vi "ZeroMQ_ReqRep_TCS.vi"() -> ()   [LabVIEW 2018]
uses:
  <vilib>/addons/zeromq/socket_type.ctl
  <vilib>/addons/zeromq/zeromq.lvlib
  <vilib>/addons/zeromq/zmq_socket.lvclass
  <vilib>/addons/zeromq/socket_options.ctl
  <vilib>/addons/zeromq/zmq_context.lvclass
panel:
  out "command":string
  in  "stop 3":bool
  out "error out 3":errorcluster
  out "reply":string
  out "error out 2":errorcluster
  out "message":string
  out "read buffer":string
  in  "stop 2":bool
  out "error out":errorcluster
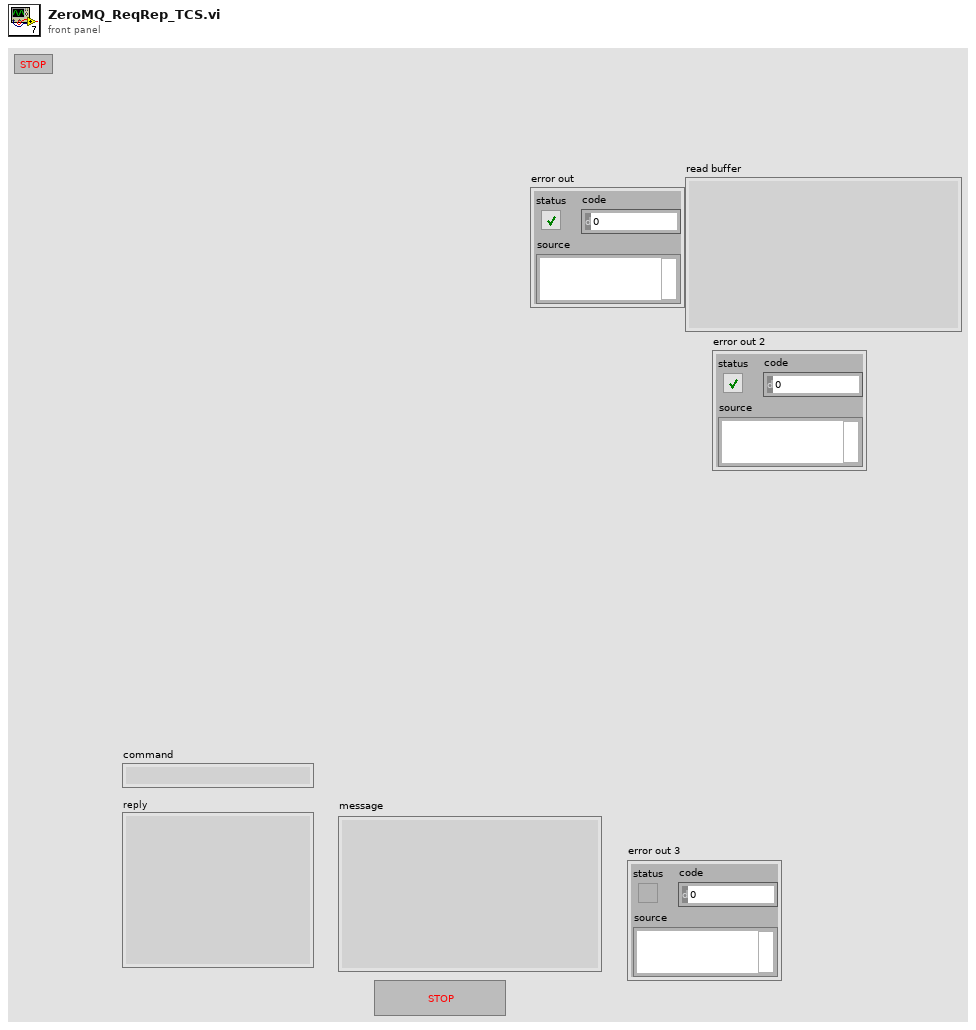
[diagram p1: front panel]
types:
  T1 = typedef "zeromq.lvlib/socket_type.ctl" = enum8{"ZMQ_PAIR", "ZMQ_PUB", "ZMQ_SUB", "ZMQ_REQ", "ZMQ_REP", "ZMQ_DEALER", "ZMQ_ROUTER", "ZMQ_PULL", "ZMQ_PUSH", "ZMQ_XPUB", "ZMQ_XSUB", "ZMQ_STREAM", "ZMQ_SERVER", "ZMQ_CLIENT", "ZMQ_RADIO", "ZMQ_DISH", "ZMQ_GATHER", "ZMQ_SCATTER", "ZMQ_DGRAM"}
  T2 = typedef "zeromq.lvlib/socket_options.ctl" = enum8{"NONE", "ZMQ_HWM", "<2>", "ZMQ_SWAP", "ZMQ_AFFINITY", "ZMQ_ROUTING_ID", "ZMQ_SUBSCRIBE", "ZMQ_UNSUBSCRIBE", "ZMQ_RATE", "ZMQ_RECOVERY_IVL", "ZMQ_MCAST_LOOP", "ZMQ_SNDBUF", "ZMQ_RCVBUF", "ZMQ_RCVMORE", "ZMQ_FD", "ZMQ_EVENTS", "ZMQ_TYPE", "ZMQ_LINGER", "ZMQ_RECONNECT_IVL", "ZMQ_BACKLOG", "ZMQ_RECOVERY_IVL_MSEC", "ZMQ_RECONNECT_IVL_MAX", "ZMQ_MAXMSGSIZE", "ZMQ_SNDHWM", "ZMQ_RCVHWM", "ZMQ_MULTICAST_HOPS", "<26>", "ZMQ_RCVTIMEO", "ZMQ_SNDTIMEO", "<29>", "<30>", "ZMQ_IPV4ONLY", "ZMQ_LAST_ENDPOINT", "ZMQ_ROUTER_MANDATORY", "ZMQ_TCP_KEEPALIVE", "ZMQ_TCP_KEEPALIVE_CNT", "ZMQ_TCP_KEEPALIVE_IDLE", "ZMQ_TCP_KEEPALIVE_INTVL", "ZMQ_TCP_ACCEPT_FILTER", "ZMQ_IMMEDIATE", "ZMQ_XPUB_VERBOSE", "ZMQ_ROUTER_RAW", "ZMQ_IPV6", "ZMQ_MECHANISM", "ZMQ_PLAIN_SERVER", "ZMQ_PLAIN_USERNAME", "ZMQ_PLAIN_PASSWORD", "ZMQ_CURVE_SERVER", "ZMQ_CURVE_PUBLICKEY", "ZMQ_CURVE_SECRETKEY", "ZMQ_CURVE_SERVERKEY", "ZMQ_PROBE_ROUTER", "ZMQ_REQ_CORRELATE", "ZMQ_REQ_RELAXED", "ZMQ_CONFLATE", "ZMQ_ZAP_DOMAIN", "ZMQ_ROUTER_HANDOVER", "ZMQ_TOS", "ZMQ_IPC_FILTER_PID", "ZMQ_IPC_FILTER_UID", "ZMQ_IPC_FILTER_GID", "ZMQ_CONNECT_ROUTING_ID", "ZMQ_GSSAPI_SERVER", "ZMQ_GSSAPI_PRINCIPAL", "ZMQ_GSSAPI_SERVICE_PRINCIPAL", "ZMQ_GSSAPI_PLAINTEXT", "ZMQ_HANDSHAKE_IVL", "<67>", "ZMQ_SOCKS_PROXY", "ZMQ_XPUB_NODROP", "ZMQ_BLOCKY", "ZMQ_XPUB_MANUAL", "ZMQ_XPUB_WELCOME_MSG", "ZMQ_STREAM_NOTIFY", "ZMQ_INVERT_MATCHING", "ZMQ_HEARTBEAT_IVL", "ZMQ_HEARTBEAT_TTL", "ZMQ_HEARTBEAT_TIMEOUT", "ZMQ_XPUB_VERBOSER", "ZMQ_CONNECT_TIMEOUT", "ZMQ_TCP_MAXRT", "ZMQ_THREAD_SAFE", "<82>", "<83>", "ZMQ_MULTICAST_MAXTPDU", "ZMQ_VMCI_BUFFER_SIZE", "ZMQ_VMCI_BUFFER_MIN_SIZE", "ZMQ_VMCI_BUFFER_MAX_SIZE", "ZMQ_VMCI_CONNECT_TIMEOUT", "ZMQ_USE_FD", "ZMQ_GSSAPI_PRINCIPAL_NAMETYPE", "ZMQ_GSSAPI_SERVICE_PRINCIPAL_NAMETYPE", "ZMQ_BINDTODEVICE", "ZMQ_ZAP_ENFORCE_DOMAIN", "ZMQ_LOOPBACK_FASTPATH", "ZMQ_METADATA", "ZMQ_MULTICAST_LOOP", "ZMQ_ROUTER_NOTIFY"}
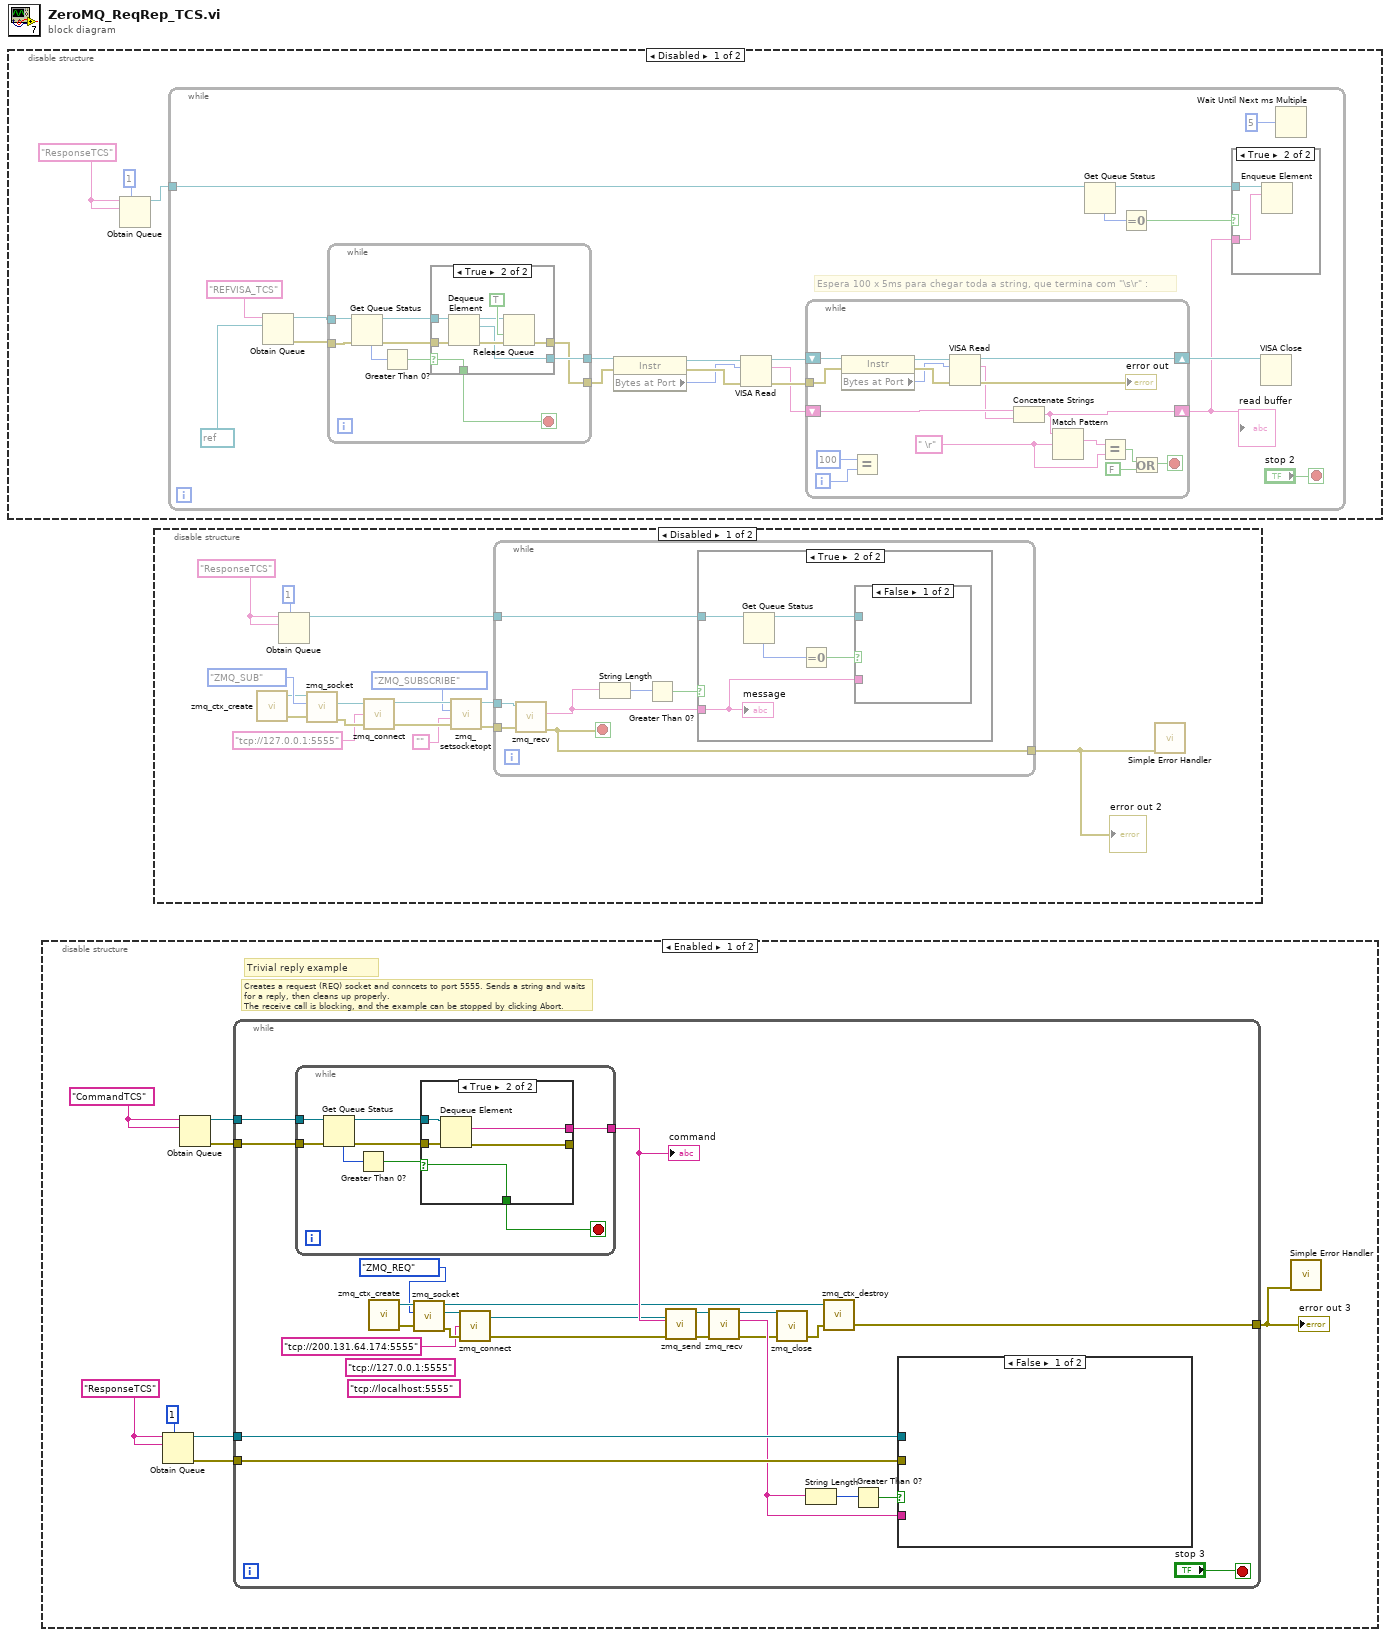
[diagram p0: block diagram]
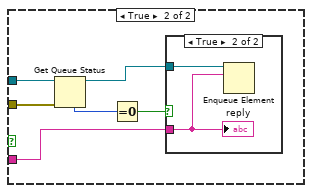
[diagram p2: hidden frame]
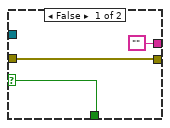
[diagram p4: hidden frame]
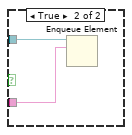
[diagram p7: hidden frame]
diagram:
  n1 = disable-structure shown="Disabled" {
    frame Disabled {
      w3 = "ResponseTCS"
      n2 = Obtain Queue(max queue size (-1, unlimited)=1, name (unnamed)=w3, element data type=w3) -> (queue out=w2:refnum<queue>)  [unwired: 2 in, 2 out]
      n3 = while {
        tunnel: w2 -> [w22]
        stop <- "stop 2" stop-if-true
        # "Espera 100 x 5ms para chegar toda a string, que termina com \"\\s\\r\" :"
        n4 = Obtain Queue(name (unnamed)="REFVISA_TCS", element data type=refnum<visa-resource-name> refnum ("VISA resource name out")) -> (queue out=w18:refnum<queue>, error out=w19:errorcluster)  [unwired: 3 in, 1 out]
        n5 = while {
          tunnel: [w46] -> w8
          tunnel: w18 -> [w45]
          tunnel: w19 -> [w44]
          tunnel: [w43] -> w7
          stop <- w47 stop-if-true
          n6 = Get Queue Status(queue=w45, error in (no error)=w44) -> (queue out=w51:refnum<queue>, error out=w50:errorcluster, # elements in queue=w48:i32)  [unwired: 1 in, 5 out]
          n7 = Greater Than 0?(x=w48) -> (x > 0?=w49:bool)
          n8 = case shown="True" w49 {
            selector: w49 -> [w53 w59]
            tunnel: w51 -> [_ w61]
            tunnel: w50 -> [w52 w60]
            tunnel: [w53 w59] -> w47
            tunnel: [_ w54] -> w46
            tunnel: [w52 w55] -> w43
            frame False {
            }
            frame True {
              n9 = Dequeue Element(queue=w61, error in (no error)=w60) -> (queue out=w57:refnum<queue>, element=w54:refnum<visa-resource-name>, error out=w56:errorcluster)  [unwired: 1 in, 1 out]
              n10 = Release Queue(queue=w57, force destroy? (F)=TRUE, error in (no error)=w56) -> (error out=w55:errorcluster)  [unwired: 2 out]
            }
          }
        }
        n11 = property class="Instr"(reference=w8, error in=w7) -> (reference out=w11:refnum<visa-resource-name>, error out=w10:errorcluster, "Bytes at Port"=w9:u32)
        n12 = VISA Read(VISA resource name=w11, byte count=w9, error in (no error)=w10) -> (VISA resource name out=w5:refnum<visa-resource-name>, read buffer=w4:string, error out=w6:errorcluster)  [unwired: 1 out]
        n13 = while {
          tunnel: w6 -> [w38]
          shift-right: [w41] -> w20
          shift-left: w5 -> [w39]
          shift-right: [w26] -> w13
          shift-left: w4 -> [w34]
          i -> [w30]
          stop <- w32 stop-if-true
          w27 = " \r" ("regular expression")
          n14 = property class="Instr"(reference=w39, error in=w38) -> (reference out=w37:refnum<visa-resource-name>, error out=w36:errorcluster, "Bytes at Port"=w35:u32)
          n15 = Equal?(x=100, y=w30) -> ()  [unwired: 1 out]
          n16 = VISA Read(VISA resource name=w37, byte count=w35, error in (no error)=w36) -> (VISA resource name out=w41:refnum<visa-resource-name>, read buffer=w33:string, error out=→"error out":errorcluster)  [unwired: 1 out]
          n17 = Concatenate Strings(w34, w33) -> (w26:string)
          n18 = Match Pattern(string=w26, regular expression=w27) -> (match substring=w40:string)  [unwired: 1 in, 3 out]
          n19 = Equal?(x=w40, y=w27) -> (x = y?=w31:bool)
          n20 = Or(x=w31, y=FALSE) -> (x .or. y?=w32:bool)
        }
        "read buffer" <- w13
        n21 = Get Queue Status(queue=w22) -> (queue out=w14:refnum<queue>, # elements in queue=w16:i32)  [unwired: 2 in, 6 out]
        n22 = Equal To 0?(x=w16) -> (x = 0?=w15:bool)
        n23 = case shown="True" w15 {
          tunnel: w14 -> [_ w25]
          tunnel: w13 -> [_ w24]
          frame False {
          }
          frame True {
            n24 = Enqueue Element(queue=w25, element=w24) -> ()  [unwired: 2 in, 3 out]
          }
        }
        n25 = VISA Close(VISA resource name=w20) -> ()  [unwired: 1 in, 1 out]
        n26 = Wait Until Next ms Multiple(millisecond multiple=u32 5) -> ()  [unwired: 1 out]
      }
    }
    frame Enabled {
    }
  }
  n27 = disable-structure shown="Enabled" {
    frame Enabled {
      w67 = "CommandTCS"
      w69 = "ResponseTCS"
      # "Creates a request (REQ) socket and conncets to port 5555. Sends a string and waits for a reply, then cleans up properly.\nThe receive call is blocking, and the example can be stopped by clicking Abort."
      # "Trivial reply example"
      n28 = Obtain Queue(max queue size (-1, unlimited)=1, name (unnamed)=w69, element data type=w69) -> (queue out=w64:refnum<queue>, error out=w63:errorcluster)  [unwired: 2 in, 1 out]
      n29 = Obtain Queue(name (unnamed)=w67, element data type=w67) -> (queue out=w66:refnum<queue>, error out=w65:errorcluster)  [unwired: 3 in, 1 out]
      n30 = while {
        tunnel: w66 -> [w91]
        tunnel: w65 -> [w90]
        tunnel: w64 -> [w88]
        tunnel: w63 -> [w87]
        tunnel: [w74] -> w62
        stop <- "stop 3" stop-if-true
        (unwired) "tcp://127.0.0.1:5555" ("endpoint")
        (unwired) "tcp://localhost:5555" ("endpoint")
        n31 = while {
          tunnel: w91 -> [w108]
          tunnel: w90 -> [w107]
          tunnel: [w103] -> w89
          stop <- w102 stop-if-true
          n32 = Get Queue Status(queue=w108, error in (no error)=w107) -> (queue out=w104:refnum<queue>, error out=w105:errorcluster, # elements in queue=w109:i32)  [unwired: 1 in, 5 out]
          n33 = Greater Than 0?(x=w109) -> (x > 0?=w106:bool)
          n34 = case shown="True" w106 {
            selector: w106 -> [w110 w113]
            tunnel: w105 -> [w112 w117]
            tunnel: w104 -> [_ w116]
            tunnel: [w112 w115] -> _
            tunnel: ["" w114] -> w103
            tunnel: [w110 w113] -> w102
            frame False {
            }
            frame True {
              n35 = Dequeue Element(queue=w116, error in (no error)=w117) -> (element=w114:string, error out=w115:errorcluster)  [unwired: 1 in, 2 out]
            }
          }
        }
        "command" <- w89
        n36 = call <vilib>:"zmq_ctx_create.vi"() -> ("error out"=w79:errorcluster, "context out"=w82:refnum<class "zmq_context.lvclass">)  [unwired: 4 in]
        n37 = call <vilib>:"zmq_socket.vi"("error in"=w79, "socket type"=socket_type."ZMQ_REQ", "context in"=w82) -> ("error out"=w81:errorcluster, "socket out"=w80:refnum<class "zmq_socket.lvclass">, "context out"=w71:refnum<class "zmq_context.lvclass">)  [unwired: 2 in]
        n38 = call <vilib>:"zmq_connect.vi"("error in"=w81, "endpoint"="tcp://200.131.64.174:5555", "socket in"=w80) -> ("error out"=w76:errorcluster, "socket out"=w77:refnum<class "zmq_socket.lvclass">)  [unwired: 1 in]
        n39 = call <vilib>:"zmq_send.vi"("error in"=w76, "data"=w89, "socket in"=w77) -> ("error out"=w92:errorcluster, "socket out"=w93:refnum<class "zmq_socket.lvclass">)  [unwired: 4 in]
        n40 = call <vilib>:"zmq_recv.vi"("error in"=w92, "socket in"=w93) -> ("error out"=w73:errorcluster, "data"=w85:string, "socket out"=w72:refnum<class "zmq_socket.lvclass">)  [unwired: 3 in, 2 out]
        n41 = call <vilib>:"zmq_close.vi"("error in"=w73, "socket"=w72) -> ("error out"=w75:errorcluster)  [unwired: 3 in]
        n42 = String Length(string=w85) -> (length=w86:i32)
        n43 = call <vilib>:"zmq_ctx_destroy.vi"("error in"=w75, "context in"=w71) -> ("error out"=w74:errorcluster)  [unwired: 3 in]
        n44 = Greater Than 0?(x=w86) -> (x > 0?=w84:bool)
        n45 = case shown="False" w84 {
          tunnel: w88 -> [_ w98]
          tunnel: w85 -> [_ w95]
          tunnel: w87 -> [_ w94]
          frame False {
          }
          frame True {
            n46 = Get Queue Status(queue=w98, error in (no error)=w94) -> (queue out=w96:refnum<queue>, # elements in queue=w99:i32)  [unwired: 1 in, 6 out]
            n47 = Equal To 0?(x=w99) -> (x = 0?=w97:bool)
            n48 = case shown="True" w97 {
              tunnel: w96 -> [_ w101]
              tunnel: w95 -> [_ w100]
              frame False {
              }
              frame True {
                n49 = Enqueue Element(queue=w101, element=w100) -> ()  [unwired: 2 in, 3 out]
                "reply" <- w100
              }
            }
          }
        }
      }
      "error out 3" <- w62
      n50 = call <vilib>:"Simple Error Handler.vi"("error in (no error)"=w62) -> ()  [unwired: 4 in, 5 out]
    }
    frame Disabled {
    }
  }
  n51 = disable-structure shown="Disabled" {
    frame Disabled {
      w120 = "ResponseTCS"
      n52 = call <vilib>:"zmq_ctx_create.vi"() -> ("error out"=w132:errorcluster, "context out"=w121:refnum<class "zmq_context.lvclass">)  [unwired: 4 in]
      n53 = Obtain Queue(max queue size (-1, unlimited)=1, name (unnamed)=w120, element data type=w120) -> (queue out=w118:refnum<queue>)  [unwired: 2 in, 2 out]
      n54 = call <vilib>:"zmq_socket.vi"("error in"=w132, "socket type"=socket_type."ZMQ_SUB", "context in"=w121) -> ("error out"=w131:errorcluster, "socket out"=w122:refnum<class "zmq_socket.lvclass">)  [unwired: 2 in, 1 out]
      n55 = call <vilib>:"zmq_connect.vi"("error in"=w131, "endpoint"="tcp://127.0.0.1:5555", "socket in"=w122) -> ("error out"=w129:errorcluster, "socket out"=w130:refnum<class "zmq_socket.lvclass">)  [unwired: 1 in]
      n56 = call <vilib>:"zmq_setsocketopt.vi"("error in"=w129, "value"="", "option"=socket_options."ZMQ_SUBSCRIBE", "socket in"=w130) -> ("error out"=w128:errorcluster, "socket out"=w127:refnum<class "zmq_socket.lvclass">)  [unwired: 2 in]
      n57 = while {
        tunnel: w127 -> [w138]
        tunnel: w128 -> [w140]
        tunnel: [w139] -> w123
        tunnel: w118 -> [w135]
        stop <- w139 stop-if-true
        n58 = call <vilib>:"zmq_recv.vi"("error in"=w140, "socket in"=w138) -> ("error out"=w139:errorcluster, "data"=w134:string)  [unwired: 3 in, 3 out]
        n59 = String Length(string=w134) -> (length=w137:i32)
        n60 = Greater Than 0?(x=w137) -> (x > 0?=w136:bool)
        n61 = case shown="True" w136 {
          tunnel: w135 -> [_ w144]
          tunnel: w134 -> [_ w141]
          frame False {
          }
          frame True {
            n62 = Get Queue Status(queue=w144) -> (queue out=w142:refnum<queue>, # elements in queue=w145:i32)  [unwired: 2 in, 6 out]
            n63 = Equal To 0?(x=w145) -> (x = 0?=w143:bool)
            n64 = case shown="False" w143 {
              tunnel: w142 -> [_ w147]
              tunnel: w141 -> [_ w146]
              frame False {
              }
              frame True {
                n65 = Enqueue Element(queue=w147, element=w146) -> ()  [unwired: 2 in, 3 out]
              }
            }
            "message" <- w141
          }
        }
      }
      "error out 2" <- w123
      n66 = call <vilib>:"Simple Error Handler.vi"("error in (no error)"=w123) -> ()  [unwired: 4 in, 5 out]
    }
    frame Enabled {
    }
  }
